vi "GetArguments.vi"() -> (0 "error out":errorcluster, 2 "output cluster":cluster{"appended path":path, "dup file":path})   [LabVIEW 2020]
uses:
  <vilib>/Utility/error.llb/Error Cluster From Error Code.vi
  <vilib>/ErrorRing/Error Ring.xnode
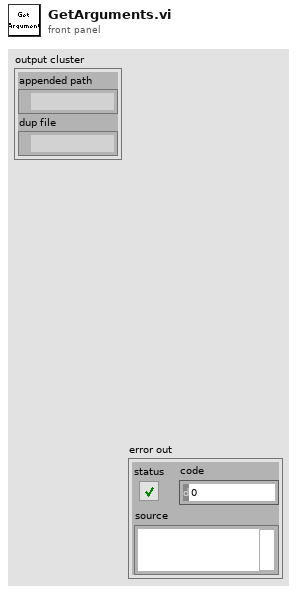
[diagram p1: front panel]
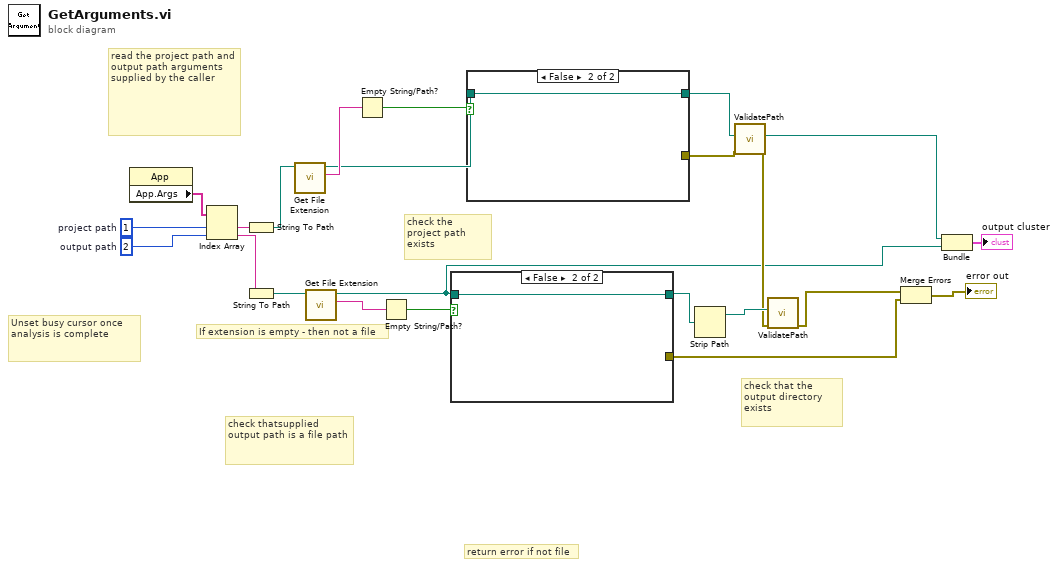
[diagram p0: block diagram]
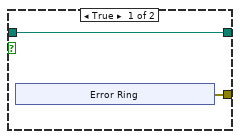
[diagram p2: hidden frame]
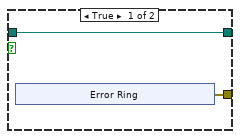
[diagram p3: hidden frame]
diagram:
  w22 = 2  # output path
  w23 = 1  # project path
  # "return error if not file"
  # "If extension is empty - then not a file"
  # "check thatsupplied output path is a file path"
  # "check that the output directory exists"
  # "check the project path exists"
  # "read the project path and output path arguments supplied by the caller"
  # "Unset busy cursor once analysis is complete"
  n1 = property class="App"() -> ("App.Args"=w21:string[])  [unwired: 2 in, 2 out]
  n2 = Index Array(array=w21, index #1=w23, index #2=w22) -> (element #1=w20:string, element #2=w9:string)
  n3 = String To Path(string=w20) -> (path=w5:path)
  n4 = String To Path(string=w9) -> (path=w18:path)
  n5 = call <vilib>:"Get File Extension.vi"("file"=w5) -> ("lowercase file extension"=w8:string, "dup file"=w6:path)  [unwired: 6 in, 3 out]
  n6 = call <vilib>:"Get File Extension.vi"("file"=w18) -> ("lowercase file extension"=w17:string, "dup file"=w10:path)  [unwired: 6 in, 3 out]
  n7 = Empty String/Path?(string/path=w8) -> (empty?=w7:bool)
  n8 = Empty String/Path?(string/path=w17) -> (empty?=w16:bool)
  n9 = case shown="False" w16 {
    tunnel: w10 -> [w25 w31]
    tunnel: [w25 w31] -> w15
    tunnel: [w24 _] -> w12
    frame True {
      n10 = xnode "Error Ring"() -> ("error out"=w24:errorcluster)
    }
    frame False {
    }
  }
  n11 = case shown="False" w7 {
    tunnel: w6 -> [w33 w39]
    tunnel: [w33 w39] -> w4
    tunnel: [w32 _] -> w3
    frame True {
      n12 = xnode "Error Ring"() -> ("error out"=w32:errorcluster)
    }
    frame False {
    }
  }
  n13 = Strip Path(path=w15) -> (stripped path=w19:path)  [unwired: 1 out]
  n14 = call "ValidatePath.vi"("error constant"=w3, "Path"=w4) -> ("error inditcator 2"=w14:errorcluster, "Path"=w2:path)  [unwired: 8 in]
  n15 = call "ValidatePath.vi"("error constant"=w14, "Path"=w19) -> ("error inditcator 2"=w13:errorcluster)  [unwired: 8 in, 1 out]
  n16 = Merge Errors(w13, w12) -> (→"error out":errorcluster)
  n17 = Bundle("Path"=w2, "dup file"=w10) -> (→"output cluster":cluster{"Path ":path, "dup file":path})  [unwired: 1 in]
